vi "DrawCircleByRadius.vi"(0 "reference in":refnum<class "LcPictureBox.lvclass">, 1 "Center":cluster{"x":sgl, "y":sgl}, 2 "Radius":sgl, 3 "Color(Black)":u32(colorbox), 4 "Alpha(100%)":dbl=100.0 min=0.0 max=100.0 format="%#_g%%", 5 "Error In":errorcluster, 7 "Fill(False)":bool, 8 "SmoothingMode(AntiAlias)":T1=enum."AntiAlias", 9 "Pen(Width=1, Solid)":T2={"Width"=1, "Style"=enum."Solid"}, 10 "StartAngle(0)":sgl, 12 "ArcSize(360)":sgl=360.0) -> (14 "reference out":refnum<class "LcPictureBox.lvclass">, 19 "Error Out":errorcluster)   [LabVIEW 2020, in "LcPictureBox.lvclass"]
uses:
  LcPictureBox.lvclass
  System.Drawing
  Pen.ctl
  SmoothingMode.ctl
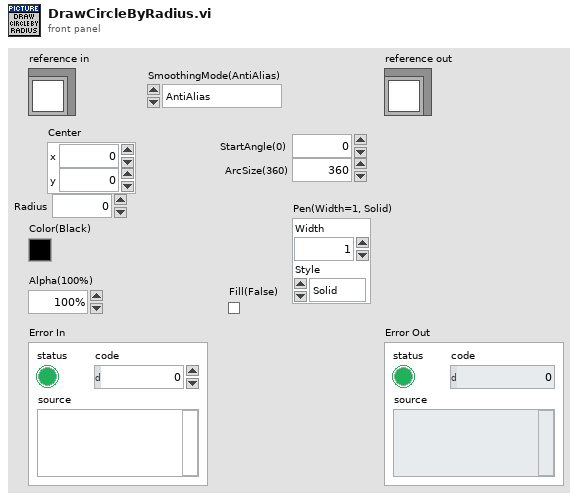
[diagram p1: front panel]
types:
  T1 = typedef "LcPictureBox.lvclass/SmoothingMode.ctl" = enum16{"None", "HighSpeed", "HighQuality", "AntiAlias"}
  T2 = typedef "LcPictureBox.lvclass/Pen.ctl" = cluster{"Width":u16, "Style":enum32{"Solid", "Dash", "Dot", "DashDot", "DashDotDot"}}
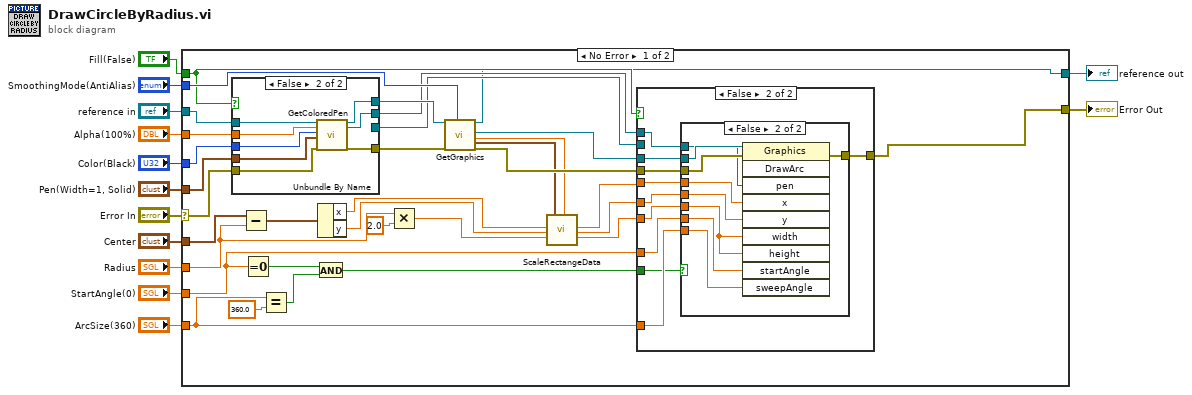
[diagram p0: block diagram]
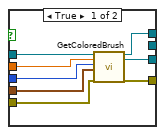
[diagram p2: hidden frame]
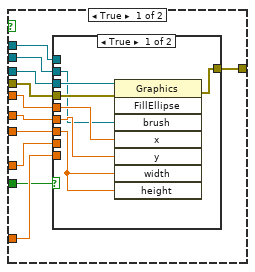
[diagram p3: hidden frame]
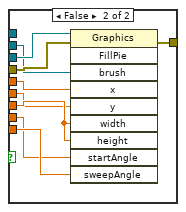
[diagram p4: hidden frame]
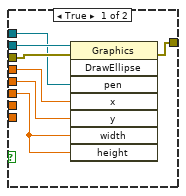
[diagram p5: hidden frame]
diagram:
  n1 = case shown="No Error" "Error In" {
    selector: "Error In" -> [w42 w117]
    tunnel: [w24 w117] -> w12
    tunnel: [w23 w116] -> w10
    tunnel: "reference in" -> [w43 w116]
    tunnel: "SmoothingMode(AntiAlias)" -> [w46 _]
    tunnel: "Color(Black)" -> [w39 _]
    tunnel: "Alpha(100%)" -> [w40 _]
    tunnel: "Pen(Width=1, Solid)" -> [w38 _]
    tunnel: "Center" -> [w27 _]
    tunnel: "Radius" -> [w25 _]
    tunnel: "StartAngle(0)" -> [w34 _]
    tunnel: "ArcSize(360)" -> [w36 _]
    tunnel: "Fill(False)" -> [w30 _]
    frame No Error {
      n2 = case shown="False" w30 {
        tunnel: [w54 w62] -> w44
        tunnel: w43 -> [w53 w61]
        tunnel: w42 -> [w52 w60]
        tunnel: [w51 w59] -> w41
        tunnel: w40 -> [w50 w58]
        tunnel: w39 -> [w49 w57]
        tunnel: w38 -> [w48 w56]
        tunnel: [_ w55] -> w37
        tunnel: [w47 _] -> w29
        frame True {
          n3 = call "GetColoredBrush.vi"("reference in"=w53, "Alpha(100%)"=w50, "Color(Black)"=w49, "Pen(Width=1, Solid)"=w48, "Error In"=w52) -> ("reference out"=w54:refnum<class "LcPictureBox.lvclass">, "SolidBrushRef"=w47:refnum<k24>, "Error Out"=w51:errorcluster)  [unwired: 12 in]
        }
        frame False {
          n4 = call "GetColoredPen.vi"("reference in"=w61, "Alpha(100%)"=w58, "Color(Black)"=w57, "Pen(Width=1, Solid)"=w56, "Error In"=w60) -> ("reference out"=w62:refnum<class "LcPictureBox.lvclass">, "PenRef"=w55:refnum<k24>, "Error Out"=w59:errorcluster)  [unwired: 12 in]
        }
      }
      n5 = Subtract(x=w27, y=w25) -> (x-y=w28:cluster{"x":sgl, "y":sgl})
      n6 = Equal To 0?(x=w34) -> (x = 0?=w33:bool)
      n7 = Equal?(x=w36, y=sgl 360.0) -> (x = y?=w32:bool)
      n8 = And(x=w33, y=w32) -> (x .and. y?=w31:bool)
      n9 = Unbundle By Name(w28) -> ("x"=w19:sgl, "y"=w17:sgl)
      n10 = Multiply(x=w25, y=sgl 2.0) -> (x*y=w15:sgl)
      n11 = call "GetGraphics.vi"("LcPictureBox in"=w44, "error in (no error)"=w41, "SmoothingMode"=w46) -> ("LcPictureBox out"=w23:refnum<class "LcPictureBox.lvclass">, "Graphics"=w22:refnum<k24>, "Scale"=w21:sgl, "Offset"=w20:cluster{"x":sgl, "y":sgl}, "error out"=w45:errorcluster)  [unwired: 12 in]
      n12 = call "ScaleRectangeData.vi"("X-In"=w19, "Y-In"=w17, "Width-In"=w15, "Offset(raw)"=w20, "Scale"=w21) -> ("X-Out"=w18:sgl, "Y-Out"=w16:sgl, "Width-Out"=w14:sgl)  [unwired: 11 in, 1 out]
      n13 = case shown="False" w30 {
        tunnel: w22 -> [w73 w99]
        tunnel: w45 -> [w72 w98]
        tunnel: w37 -> [w71 w97]
        tunnel: w14 -> [w70 w96]
        tunnel: w16 -> [w69 w95]
        tunnel: w18 -> [w68 w94]
        tunnel: [w67 w93] -> w24
        tunnel: w36 -> [w66 w92]
        tunnel: w34 -> [w65 w91]
        tunnel: w31 -> [w64 w90]
        tunnel: w29 -> [w63 _]
        frame True {
          n14 = case shown="True" w64 {
            tunnel: w73 -> [w80 w89]
            tunnel: w72 -> [w79 w88]
            tunnel: w71 -> [_ _]
            tunnel: w70 -> [w75 w87]
            tunnel: w69 -> [w78 w86]
            tunnel: w68 -> [w77 w85]
            tunnel: [w76 w84] -> w67
            tunnel: w66 -> [_ w83]
            tunnel: w65 -> [_ w82]
            tunnel: w63 -> [w74 w81]
            frame True {
              n15 = invoke class="Graphics" method="FillEllipse"(reference=w80, error in=w79, "brush"=w74, "x"=w77, "y"=w78, "width"=w75, "height"=w75) -> (error out=w76:errorcluster)  [unwired: 1 in, 7 out]
            }
            frame False {
              n16 = invoke class="Graphics" method="FillPie"(reference=w89, error in=w88, "brush"=w81, "x"=w85, "y"=w86, "width"=w87, "height"=w87, "startAngle"=w82, "sweepAngle"=w83) -> (error out=w84:errorcluster)  [unwired: 1 in, 9 out]
            }
          }
        }
        frame False {
          n17 = case shown="False" w90 {
            tunnel: w99 -> [w106 w115]
            tunnel: w98 -> [w105 w114]
            tunnel: w97 -> [w104 w113]
            tunnel: w96 -> [w100 w112]
            tunnel: w95 -> [w103 w111]
            tunnel: w94 -> [w102 w110]
            tunnel: [w101 w109] -> w93
            tunnel: w92 -> [_ w108]
            tunnel: w91 -> [_ w107]
            frame True {
              n18 = invoke class="Graphics" method="DrawEllipse"(reference=w106, error in=w105, "pen"=w104, "x"=w102, "y"=w103, "width"=w100, "height"=w100) -> (error out=w101:errorcluster)  [unwired: 1 in, 7 out]
            }
            frame False {
              n19 = invoke class="Graphics" method="DrawArc"(reference=w115, error in=w114, "pen"=w113, "x"=w110, "y"=w111, "width"=w112, "height"=w112, "startAngle"=w107, "sweepAngle"=w108) -> (error out=w109:errorcluster)  [unwired: 1 in, 9 out]
            }
          }
        }
      }
    }
    frame Error {
    }
  }
  "Error Out" <- w12
  "reference out" <- w10
